vi "Event Identifier.vi"(8 "error in (no error)":errorcluster, 11 "Extension in":refnum<class "Custom ID.lvclass">) -> (0 "error out":errorcluster, 2 "Event Identifier":string)   [LabVIEW 2024, in "serenial.io-ase.test.lvlib" / "Custom ID.lvclass"]
uses:
  Custom ID.lvclass
  Custom ID.lvclass/Custom ID.ctl
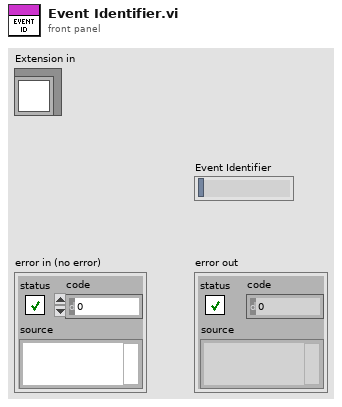
[diagram p1: front panel]
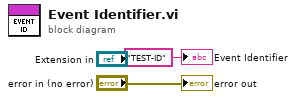
[diagram p0: block diagram]
diagram:
  "error out" <- "error in (no error)"
  "Event Identifier" <- "TEST-ID" ("Event Identifier")
